vi "Decode Constant.vi"(8 "error in (no error)":errorcluster, 11 "JSON":string) -> (0 "error out":errorcluster, 2 "Remaining JSON":string, 3 "Value":variant)   [LabVIEW 2019, in "JSON.lvlib"]
doc: "Decodes JSON constants: False, True, NaN, Null\n\nCreated by: Ryan Pacini"
uses:
  JSON.lvlib
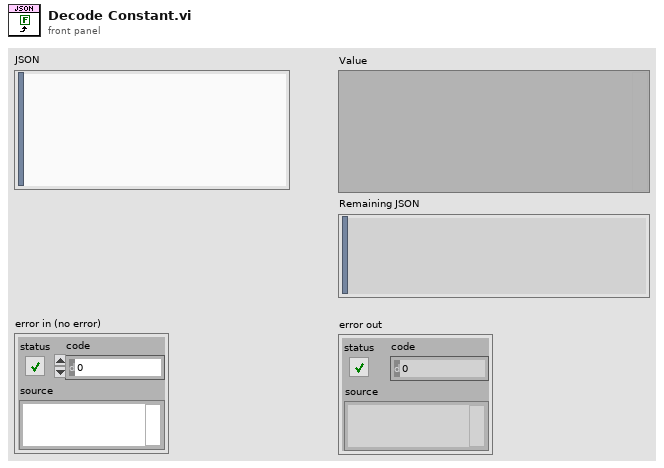
[diagram p1: front panel]
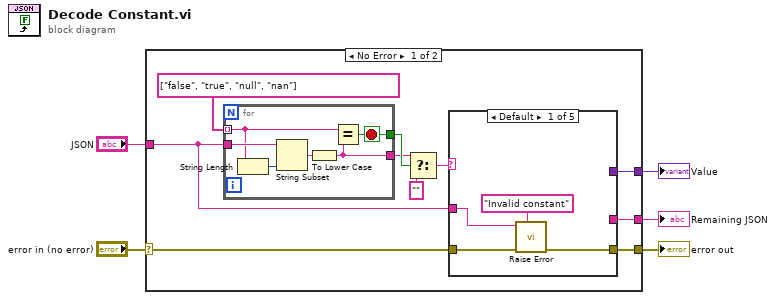
[diagram p0: block diagram]
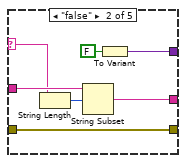
[diagram p2: hidden frame]
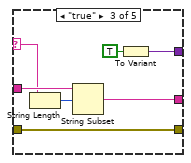
[diagram p3: hidden frame]
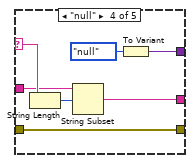
[diagram p4: hidden frame]
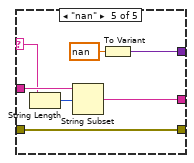
[diagram p5: hidden frame]
diagram:
  n1 = case shown="No Error" "error in (no error)" {
    selector: "error in (no error)" -> [w14 w54]
    tunnel: "JSON" -> [w7 _]
    tunnel: [w15 w54] -> w4
    tunnel: [w9 _] -> w2
    tunnel: [w6 _] -> w1
    frame No Error {
      n2 = for {
        tunnel: w7 -> [w53]
        tunnel: string[] ["false", "true", "null", "nan"] -> [w51] mode=indexing
        tunnel: [w49] -> w11
        tunnel: [w48] -> w12
        stop <- w48 stop-if-true
        n3 = String Length(string=w51) -> (length=w52:i32)
        n4 = String Subset(string=w53, length (rest)=w52) -> (substring=w50:string)  [unwired: 1 in]
        n5 = To Lower Case(string=w50) -> (all lower case string=w49:string)
        n6 = Equal?(x=w51, y=w49) -> (x = y?=w48:bool)
      }
      n7 = Select(t=w11, s=w12, f="") -> (s? t:f=w8:string)
      n8 = case shown="Default" w8 {
        selector: w8 -> [_ w20 w28 w38 w41]
        tunnel: [w17 w26 w33 w40 w47] -> w15
        tunnel: w14 -> [w19 w26 w33 w40 w47]
        tunnel: [_ w24 w31 w34 w45] -> w9
        tunnel: w7 -> [w18 w22 w30 w37 w42]
        tunnel: [_ w21 w29 w36 w43] -> w6
        frame Default {
          n9 = call "Raise Error.vi"("message"="Invalid constant" ("error message (\"\")"), "error in (no error)"=w19, "json"=w18) -> ("error out"=w17:errorcluster)  [unwired: 8 in]
        }
        frame "false" {
          n10 = String Length(string=w20) -> (length=w23:i32)
          n11 = String Subset(string=w22, offset (0)=w23) -> (substring=w21:string)  [unwired: 1 in]
          n12 = To Variant(anything=FALSE) -> (Variant=w24:variant)
        }
        frame "true" {
          n13 = String Length(string=w28) -> (length=w27:i32)
          n14 = String Subset(string=w30, offset (0)=w27) -> (substring=w29:string)  [unwired: 1 in]
          n15 = To Variant(anything=TRUE) -> (Variant=w31:variant)
        }
        frame "null" {
          n16 = String Length(string=w38) -> (length=w39:i32)
          n17 = String Subset(string=w37, offset (0)=w39) -> (substring=w36:string)  [unwired: 1 in]
          n18 = To Variant(anything=enum8{"null"}."null") -> (Variant=w34:variant)
        }
        frame "nan" {
          n19 = String Length(string=w41) -> (length=w44:i32)
          n20 = String Subset(string=w42, offset (0)=w44) -> (substring=w43:string)  [unwired: 1 in]
          n21 = To Variant(anything=nan) -> (Variant=w45:variant)
        }
      }
    }
    frame Error {
    }
  }
  "error out" <- w4
  "Value" <- w2
  "Remaining JSON" <- w1
